vi "Get DO Status - Single.vi"(0 "reference in":refnum<class "DO.lvclass">, 2 "DO Channel Number (Zero Based)":i32, 5 "error in (no error)":errorcluster) -> (14 "reference out":refnum<class "DO.lvclass">, 18 "DO Channel Status":bool, 19 "error out":errorcluster)   [LabVIEW 2017, in "DO.lvclass"]
uses:
  DO.lvclass
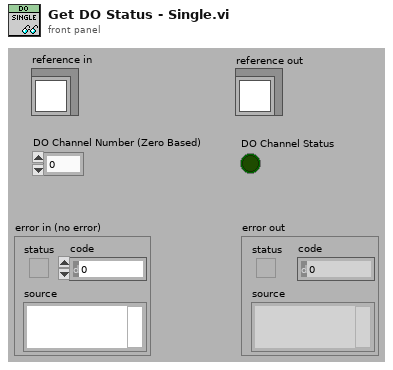
[diagram p1: front panel]
types:
  T1 = typedef "DO.lvclass/ObjectAttributes.ctl" = cluster{"DO Task":refnum<k21>, "DO Module Names (NI-Max Name)":string[], "Number of Channels Per DO Module":i32[], "DO Status":bool[], "Number of DO Modules":u32, "DO Status to Set":bool[], "DO On/Off Status":bool, "DO VI Reference":refnum<vi>, "Number of Total DO Channels":u32}
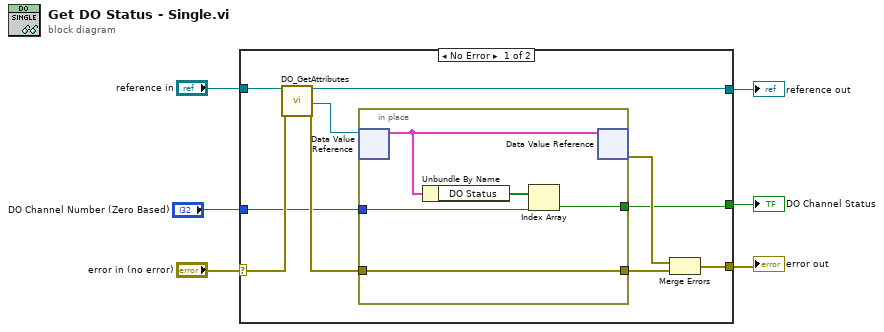
[diagram p0: block diagram]
diagram:
  n1 = case shown="No Error" "error in (no error)" {
    selector: "error in (no error)" -> [w15 w23]
    tunnel: [w12 w23] -> w5
    tunnel: [w13 w22] -> w3
    tunnel: "reference in" -> [w16 w22]
    tunnel: "DO Channel Number (Zero Based)" -> [w8 _]
    tunnel: [w7 _] -> w1
    frame No Error {
      n2 = call "DO_GetAttributes.vi"("reference in"=w16, "error in (no error)"=w15) -> ("reference out"=w13:refnum<class "DO.lvclass">, "DataRef"=w11:refnum<data-value>, "error out"=w10:errorcluster)  [unwired: 14 in, 1 out]
      n3 = in-place {
        in-place-border: w10 -> [w21]
        in-place-border: [w21] -> w9
        in-place-border: w8 -> [w18]
        in-place-border: [w17] -> w7
        n4 = in-place-dvr #1(w11) -> (w20:T1)  [unwired: 1 out]
        n5 = Unbundle By Name(w20) -> ("DO Status"=w19:bool[])
        n6 = Index Array(array=w19, index=w18) -> (element=w17:bool)
        n7 = in-place-dvr #1(w20) -> (w14:errorcluster)  [unwired: 1 out]
      }
      n8 = Merge Errors(w14, w9) -> (w12:errorcluster)
    }
    frame Error {
    }
  }
  "error out" <- w5
  "reference out" <- w3
  "DO Channel Status" <- w1
